vi "scarica.vi"() -> ()   [LabVIEW 2018]
uses:
  Control 1.ctl
  Control 2.ctl
  Control 3.ctl
  Control 4.ctl
panel:
  in  "Slide":T1=1.708860759493671 scale=0.0..10.0
  out "XY Graph":cluster{"Array":dbl[], dbl[]}(graph)
  in  "N":T2=100.0
  in  "fine":T3=10.0 min=0.0
  in  "inizio":T4 min=0.0
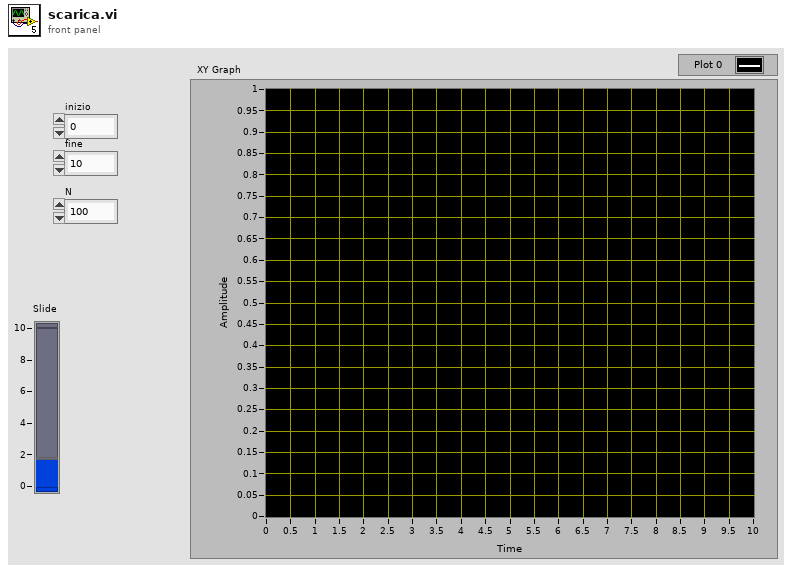
[diagram p1: front panel]
types:
  T1 = typedef "Control 4.ctl" = dbl
  T2 = typedef "Control 3.ctl" = dbl
  T3 = typedef "Control 2.ctl" = dbl
  T4 = typedef "Control 1.ctl" = dbl
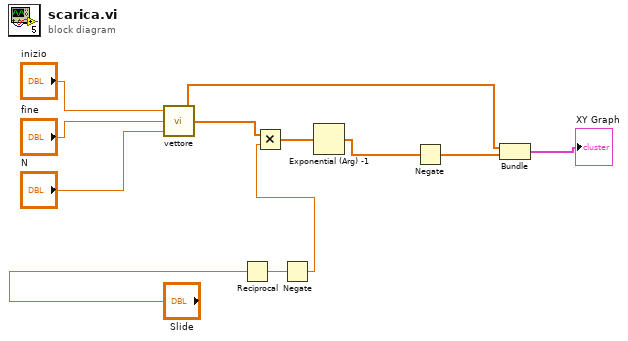
[diagram p0: block diagram]
diagram:
  n1 = call "vettore.vi"("n"="N", "fine"="fine", "inizio"="inizio") -> ("Array"=w4:dbl[])
  n2 = Reciprocal(x="Slide") -> (1/x=w8:T1)
  n3 = Negate(x=w8) -> (-x=w7:T1)
  n4 = Multiply(x=w4, y=w7) -> (x*y=w6:T1[])
  n5 = Exponential (Arg) -1(1:w6) -> (0:w5:T1[])
  n6 = Negate(x=w5) -> (-x=w3:T1[])
  n7 = Bundle("Array"=w4, w3) -> (→"XY Graph":cluster{"Array":dbl[], T1[]})  [unwired: 1 in]
